vi "Do Something Ex.vi"() -> ()   [LabVIEW 2020]
uses:
  Type.ctl
  ByRef Add/ByRef Add.lvclass
  C:/dev/LabVIEW/ByRef & Callbacks/ByRef Base/ByRef Base.lvclass
  ByRef Mul/ByRef Mul.lvclass
  ByRef Base/ByRef Base.lvclass
panel:
  in  "Type":T1
  out "Get Number":dbl
  out "Stop":bool
  in  "Do Something":bool
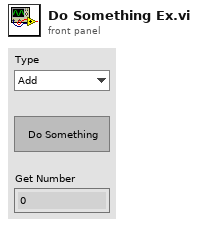
[diagram p1: front panel]
types:
  T1 = typedef "Type.ctl" = enum16{"Add", "Mul"}
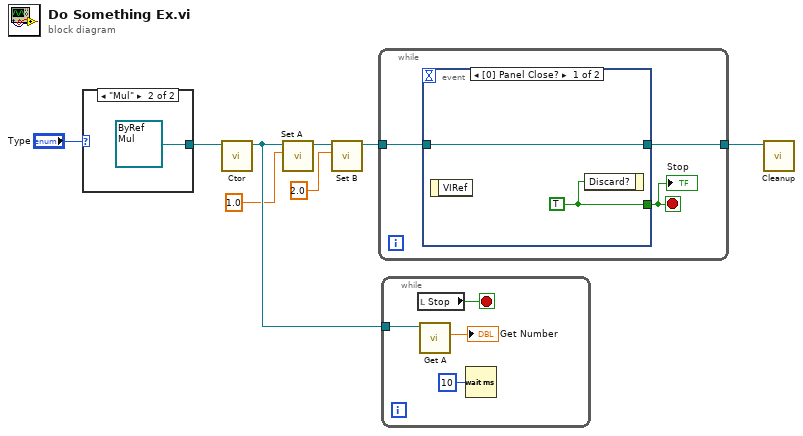
[diagram p0: block diagram]
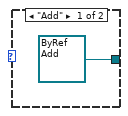
[diagram p2: hidden frame]
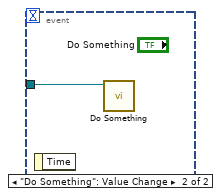
[diagram p3: hidden frame]
diagram:
  n1 = case shown="\"Mul\"" "Type" {
    tunnel: [refnum<class "ByRef Add.lvclass"> refnum ("ByRef Add.lvclass") refnum<class "ByRef Mul.lvclass"> refnum ("ByRef Mul.lvclass")] -> w1
    frame "Add" {
    }
    frame "Mul" {
    }
  }
  n2 = call-dynamic "Ctor.vi"("ByRef Base in"=w1) -> ("ByRef Base out"=w7:refnum<class "ByRef Base.lvclass">)  [unwired: 9 in, 1 out]
  n3 = call "Set A.vi"("Numeric"=1.0 ("To Add"), "ByRef Base in"=w7) -> ("ByRef Base out"=w5:refnum<class "ByRef Base.lvclass">)  [unwired: 8 in, 1 out]
  n4 = call "Set B.vi"("B"=2.0, "ByRef Base in"=w5) -> ("ByRef Base out"=w3:refnum<class "ByRef Base.lvclass">)  [unwired: 8 in, 1 out]
  n5 = while {
    tunnel: w3 -> [w12]
    tunnel: [w11] -> w8
    stop <- w13 stop-if-true
    n6 = event shown="[0] Panel Close?" {
      selector: _ -> [_ _]
      dyn-events: _ -> [_ _]
      timeout: _ -> [_ _]
      tunnel: [w14 _] -> w13
      tunnel: w12 -> [w15 w16]
      tunnel: [w15 _] -> w11
      event Panel Close? {
        w14 = TRUE
        n7 = event-data() -> ()  [unwired: 1 in, 1 out]
        n8 = event-data("Discard?"=w14) -> ()  [unwired: 1 in, 1 out]
      }
      event "Do Something": Value Change {
        n9 = event-data() -> ()  [unwired: 1 in, 1 out]
        n10 = call-dynamic "Do Something.vi"("ByRef Base in"=w16) -> ()  [unwired: 9 in, 2 out]
      }
    }
    "Stop" <- w13
  }
  n11 = while {
    tunnel: w7 -> [w19]
    stop <- w20 stop-if-true
    n12 = local read "Stop"() -> (w20:bool)
    n13 = call "Get A.vi"("ByRef Base in"=w19) -> ("Numeric"=→"Get Number":dbl)  [unwired: 8 in, 2 out]
    n14 = Wait (ms)(milliseconds to wait=u32 10) -> ()  [unwired: 1 out]
  }
  n15 = call-dynamic "Cleanup.vi"("ByRef Base in"=w8) -> ()  [unwired: 10 in, 1 out]
